vi "myRIO_BRig_Host_TCP_parseCmd_selectResponse__subunit1.vi"(8 "input_arrayUnknown":i32[][](array[numeric]), 9 "input_idxUnknown":i32, 10 "input_countCmd":i32, 11 "input_strCmd":string) -> (0 "output_countTrial":i32, 1 "output_L/R":i32, 2 "output_iTrial":i32, 3 "output_iBlock":i32, 4 "output_idxUnknown":i32, 5 "output_response":i32, 6 "output_arrayUnknown":i32[][](array[numeric]))   [LabVIEW 2014]
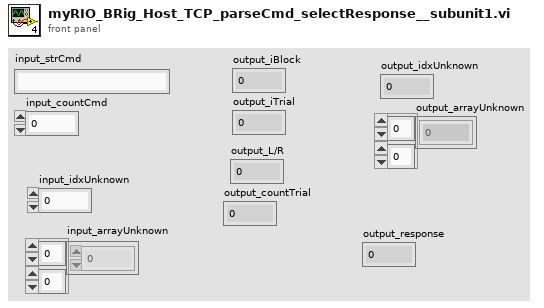
[diagram p1: front panel]
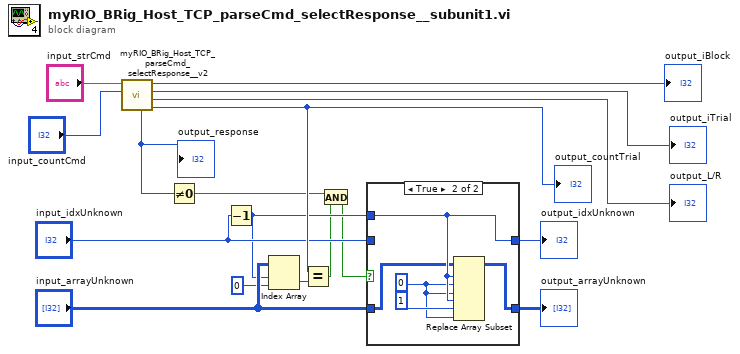
[diagram p0: block diagram]
diagram:
  n1 = call "myRIO_BRig_Host_TCP_parseCmd_selectResponse__v2.vi"("input_countCmd"="input_countCmd", "input_strCmd"="input_strCmd") -> ("output_countTrial"=w13:i32, "output_L/R"=→"output_L/R":i32, "output_iTrial"=→"output_iTrial":i32, "output_iBlock"=→"output_iBlock":i32, "output_response"=w4:i32)  [unwired: 5 in]
  "output_countTrial" <- w13
  "output_response" <- w4
  n2 = Not Equal To 0?(x=w4) -> (x != 0?=w1:bool)
  n3 = Decrement(x="input_idxUnknown") -> (x-1=w5:i32)
  n4 = Index Array(array="input_arrayUnknown", index (row)=w5, index (col)=0 ("disabled index (col)")) -> (element=w6:i32)
  n5 = Equal?(x=w13, y=w6) -> (x = y?=w3:bool)
  n6 = And(x=w1, y=w3) -> (x .and. y?=w2:bool)
  n7 = case shown="True" w2 {
    tunnel: "input_arrayUnknown" -> [w19 w21]
    tunnel: [w19 w20] -> w11
    tunnel: [w18 w23] -> w12
    tunnel: "input_idxUnknown" -> [w18 _]
    tunnel: w5 -> [_ w23]
    frame False {
    }
    frame True {
      w22 = 0 ("new element/subarray")
      n8 = Replace Array Subset(array=w21, new element #1=w22, index (row) #1=w23, index (col) #1=w22, new element #2=w22, index (row) #2=w23, index (col) #2=1 ("new element/subarray")) -> (w20:i32[][])
    }
  }
  "output_idxUnknown" <- w12
  "output_arrayUnknown" <- w11
